vi "getfromserver.vi"(1 "Line Number":string, 2 "Direction":string, 3 "Stop ID":string) -> (0 "Result Body":string)   [LabVIEW 2023]
uses:
  <vilib>/httpClient/LabVIEWHTTPClient.lvlib
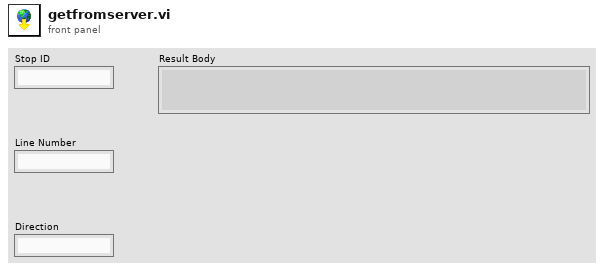
[diagram p1: front panel]
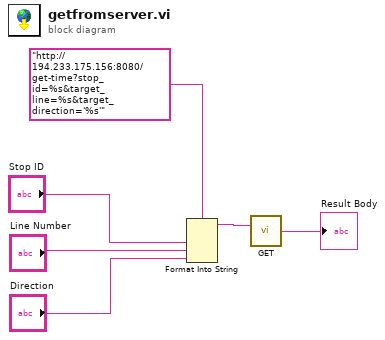
[diagram p0: block diagram]
diagram:
  n1 = Format Into String(format string="http://194.233.175.156:8080/get-time?stop_id=%s&target_line=%s&target_direction='%s'" ("url"), "Stop ID", "Line Number", "Direction") -> (resulting string=w3:string)  [unwired: 2 in, 1 out]
  n2 = call <vilib>:"GET.vi"("url"=w3) -> ("body"=→"Result Body":string)  [unwired: 11 in, 3 out]
